vi "deserialize (Messages-Ballard).vi"(11 "data in":string[][](array[string])) -> (3 "messages":map{string, T1}[](array[numeric]))   [LabVIEW 2020]
uses:
  _controls/aim1553_messages.ctl
  _controls/ballard1553_messages.ctl
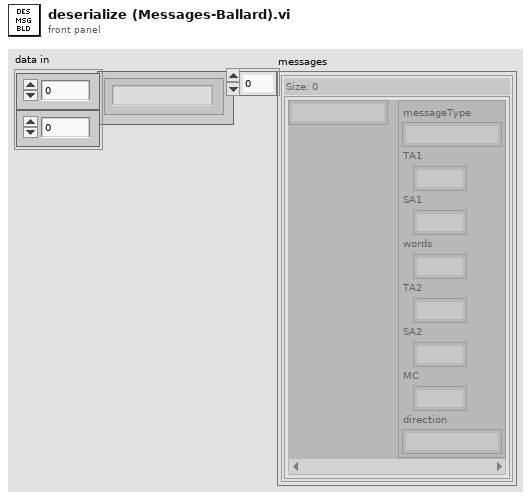
[diagram p1: front panel]
types:
  T1 = typedef "aim1553_messages.ctl" = cluster{"messageType":string, "TA1":i32, "SA1":i32, "words":i32, "TA2":i32, "SA2":i32, "MC":i32, "direction":string}
  T2 = typedef "ballard1553_messages.ctl" = cluster{"messageType":string, "TA1":i32, "SA1":i32, "words":i32, "TA2":i32, "SA2":i32, "MC":i32, "direction":string}
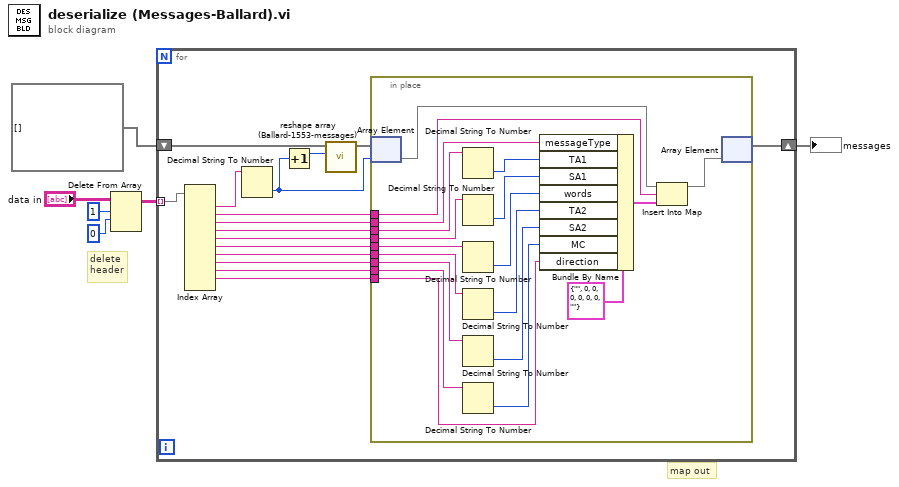
[diagram p0: block diagram]
diagram:
  # "delete\nheader"
  # "map out"
  n1 = Delete From Array(array="data in", length=1, index (row)=0) -> (array with subset deleted=w1:string[][])  [unwired: 1 in, 1 out]
  n2 = for {
    tunnel: w1 -> [w22] mode=indexing
    shift-right: [w8] -> w5
    shift-left: map{string, T2}[] [] ("map") -> [w11]
    n3 = Index Array(array=w22) -> (element #1=w12:string, element #2=w21:string, element #3=w20:string, element #4=w19:string, element #5=w18:string, element #6=w17:string, element #7=w16:string, element #8=w15:string, element #9=w14:string, element #10=w13:string)  [unwired: 11 in, 1 out]
    n4 = Decimal String To Number(string=w12) -> (number=w9:i32)  [unwired: 2 in, 1 out]
    n5 = Increment(x=w9) -> (x+1=w7:i32)
    n6 = call "reshape array (Ballard-1553-messages).vi"("index requested"=w7, "messages in"=w11) -> ("messages out"=w10:map{string, T1}[])  [unwired: 9 in]
    n7 = in-place {
      in-place-border: w21 -> [w39]
      in-place-border: w20 -> [w38]
      in-place-border: w19 -> [w37]
      in-place-border: w18 -> [w35]
      in-place-border: w17 -> [w34]
      in-place-border: w16 -> [w31]
      in-place-border: w15 -> [w30]
      in-place-border: w14 -> [w29]
      in-place-border: w13 -> [w28]
      n8 = in-place-array #1(w10, w9) -> (w24:map{string, T1})
      n9 = Decimal String To Number(string=w37) -> (number=w36:i32)  [unwired: 2 in, 1 out]
      n10 = Decimal String To Number(string=w35) -> (number=w33:i32)  [unwired: 2 in, 1 out]
      n11 = Decimal String To Number(string=w34) -> (number=w32:i32)  [unwired: 2 in, 1 out]
      n12 = Decimal String To Number(string=w31) -> (number=w27:i32)  [unwired: 2 in, 1 out]
      n13 = Decimal String To Number(string=w30) -> (number=w26:i32)  [unwired: 2 in, 1 out]
      n14 = Decimal String To Number(string=w29) -> (number=w25:i32)  [unwired: 2 in, 1 out]
      n15 = Bundle By Name(cluster=T2 {"messageType"="", "TA1"=0, "SA1"=0, "words"=0, "TA2"=0, "SA2"=0, "MC"=0, "direction"=""}, "messageType"=w38, "TA1"=w36, "SA1"=w33, "words"=w32, "TA2"=w27, "SA2"=w26, "MC"=w25, "direction"=w28) -> (w40:T2)
      n16 = Insert Into Map(map in=w24, key=w39, value=w40) -> (map out=w23:map{string, T1})  [unwired: 2 out]
      n17 = in-place-array #1(w23) -> (w8:map{string, T1}[])  [unwired: 1 out]
    }
  }
  "messages" <- w5
